vi "ASK_Picturecode.vi"(8 "picture_model":i32, 9 "picture_path":string, 11 "PathIn":path) -> (0 "error out":errorcluster caption="错误输出", 2 "Origin_Bit":dbl[](array[numeric]) format="%#_13g", 3 "PathOut":path, 4 "N":dbl, 5 "M":dbl)   [LabVIEW 2015]
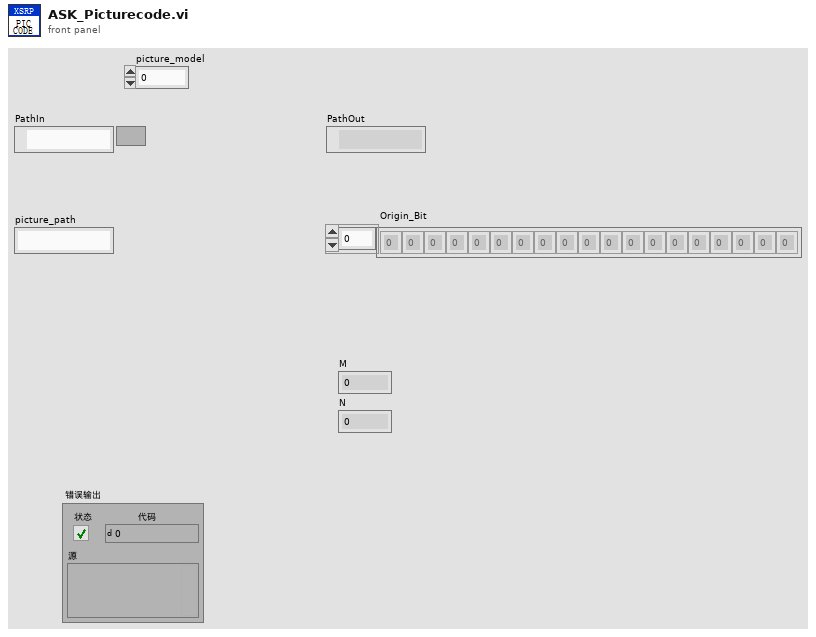
[diagram p1: front panel]
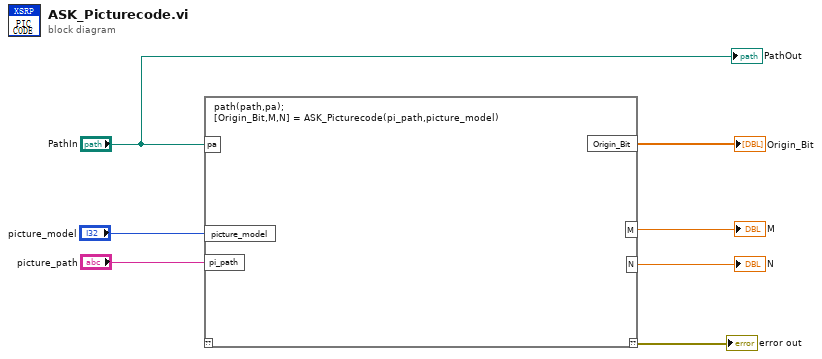
[diagram p0: block diagram]
diagram:
  n1 = script code="path(path,pa);\n[Origin_Bit,M,N] = ASK_Picturecode(pi_path,picture_model)"("pa"="PathIn", "pi_path"="picture_path", "picture_model"="picture_model") -> ("??"=→"error out":errorcluster, "Origin_Bit"=→"Origin_Bit":dbl[], "M"=→"M":dbl, "N"=→"N":dbl)  [unwired: 1 in]
  "PathOut" <- "PathIn"
